vi "Find User Added Node Type.vi"(10 "Node Tag Name":string) -> (2 "UserAddedNodeType":T1(ring))   [LabVIEW 2025]
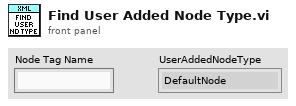
[diagram p1: front panel]
types:
  T1 = enum16{"DefaultNode", "DynamicNode", "Properties", "Section"}
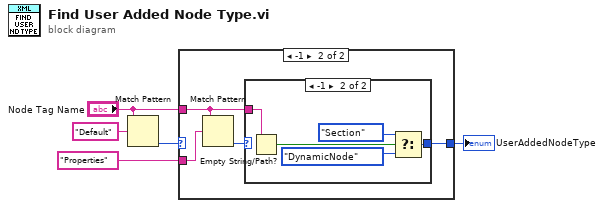
[diagram p0: block diagram]
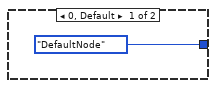
[diagram p2: hidden frame]
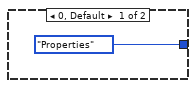
[diagram p3: hidden frame]
diagram:
  n1 = Match Pattern(string="Node Tag Name", regular expression="Default") -> (offset past match=w4:i32)  [unwired: 1 in, 3 out]
  n2 = case shown="-1" w4 {
    tunnel: [T1."DefaultNode" w8] -> w1
    tunnel: "Node Tag Name" -> [_ w7]
    tunnel: "Properties" ("regular expression") -> [_ w10]
    frame 0, Default {
    }
    frame -1 {
      n3 = Match Pattern(string=w7, regular expression=w10) -> (offset past match=w9:i32)  [unwired: 1 in, 3 out]
      n4 = case shown="-1" w9 {
        tunnel: [T1."Properties" w13] -> w8
        tunnel: w7 -> [_ w12]
        frame 0, Default {
        }
        frame -1 {
          n5 = Empty String/Path?(string/path=w12) -> (empty?=w16:bool)
          n6 = Select(t=T1."Section", s=w16, f=T1."DynamicNode") -> (s? t:f=w13:T1)
        }
      }
    }
  }
  "UserAddedNodeType" <- w1
